vi "View Launcher.vi"(8 "error in (no error)":errorcluster, 11 "Max UUTs to Store":i32) -> (0 "error out":errorcluster)   [LabVIEW 2019, in "STS_LTRV.lvlib"]
uses:
  STS_LTRV.lvlib
  TypeDefs/Event Handler/Operation.ctl
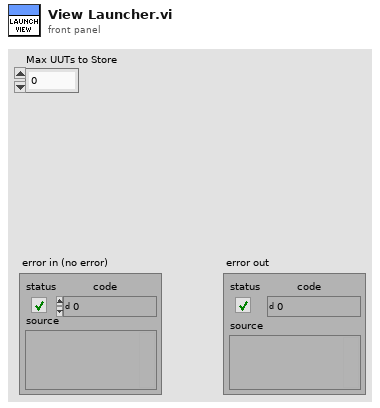
[diagram p1: front panel]
types:
  T1 = typedef "STS_LTRV.lvlib/Operation.ctl" = enum16{"Initilize", "Get Reference", "Publish", "Destroy"}
  T2 = enum32{"Bad", "Idle", "Run top level", "Running"}
  T3 = enum32{"Invalid", "Standard", "Closed", "Hidden", "Minimized", "Maximized"}
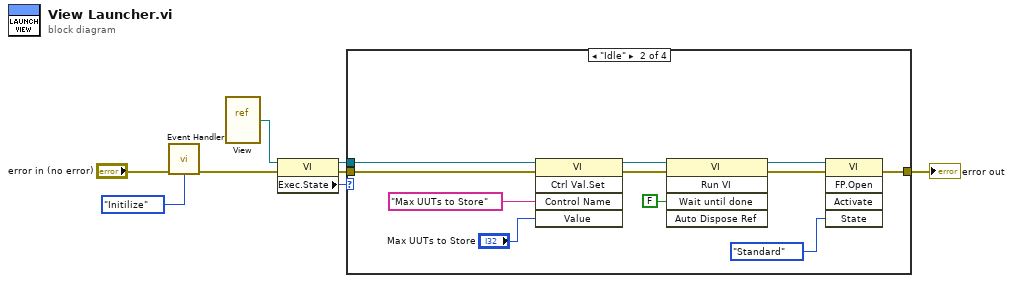
[diagram p0: block diagram]
diagram:
  n1 = call "Event Handler.vi"("error in (no error)"="error in (no error)", "Operation"=Operation."Initilize") -> ("error out"=w2:errorcluster)  [unwired: 12 in, 1 out]
  n2 = vi-ref "View.vi"() -> (w8:refnum<vi>)
  n3 = property class="VI"(reference=w8, error in=w2) -> (reference out=w5:refnum<vi>, error out=w7:errorcluster, "Exec.State"=w6:T2)
  n4 = case shown="\"Idle\"" w6 {
    tunnel: w7 -> [w9 w15 w21 w22]
    tunnel: w5 -> [_ w14 _ _]
    tunnel: [w9 w16 w21 w22] -> w4
    frame "Bad", Default {
    }
    frame "Idle" {
      n5 = invoke class="VI" method="Ctrl Val.Set"(reference=w14, error in=w15, "Control Name"="Max UUTs to Store", "Value"="Max UUTs to Store") -> (reference out=w13:refnum<vi>, error out=w12:errorcluster)  [unwired: 1 in, 3 out]
      n6 = invoke class="VI" method="Run VI"(reference=w13, error in=w12, "Wait until done"=FALSE ("Wait Until Done")) -> (reference out=w18:refnum<vi>, error out=w19:errorcluster)  [unwired: 2 in, 3 out]
      n7 = invoke class="VI" method="FP.Open"(reference=w18, error in=w19, "State"=T3."Standard") -> (error out=w16:errorcluster)  [unwired: 2 in, 4 out]
    }
    frame "Run top level" {
    }
    frame "Running" {
    }
  }
  "error out" <- w4
